vi "STOP.vi"(0 "System no.":i32=1 min=1 max=4 step=1, 5 "error in":errorcluster) -> (19 "error out":errorcluster)   [LabVIEW 2020]
doc: "Stops single motion (to stop fast scan routines use #24). \n\nF-206, M-8X0: Only for GCS syntax version = GCS 1.0 (check with CSV?.vi. If CSV?.vi is not supported, syntax version is GCS 1.0). For GCS 2.0 or higher, use STP.vi instead."
panel:
  # "Stop single motion (for fast scan routines use #24). New command: STP"
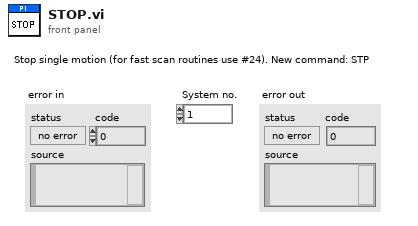
[diagram p1: front panel]
types:
  T1 = enum16{"Disable error check", "Force error check", "Use global settings"}
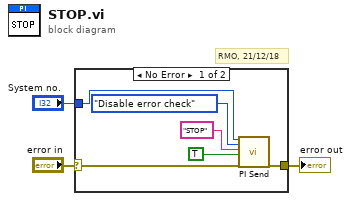
[diagram p0: block diagram]
diagram:
  # "RMO, 21/12/18"
  n1 = case shown="No Error" "error in" {
    selector: "error in" -> [w5 w10]
    tunnel: [w9 w10] -> w3
    tunnel: "System no." -> [w6 _]
    frame No Error {
      n2 = call "PI Send.vi"("System no."=w6, "Error check settings"=T1."Disable error check", "String to send"="STOP", "Attach termination char.?"=TRUE ("Attach Linefeed?"), "error in"=w5) -> ("error out"=w9:errorcluster)  [unwired: 1 in, 13 out]
    }
    frame Error {
    }
  }
  "error out" <- w3
